vi "PH_Periodic_Sequencer.read DB.vi"(0 "i ref in":refnum<vi>, 5 "error in (no error)":errorcluster) -> (14 "i ref out":refnum<vi>, 19 "error out":errorcluster)   [LabVIEW 2009]
doc: "This VI reads out information from the database and stores it to own attributes."
uses:
  PH_Periodic_Sequencer.lvlib
  CSCore/BaseProcess/BaseProcess.lvlib
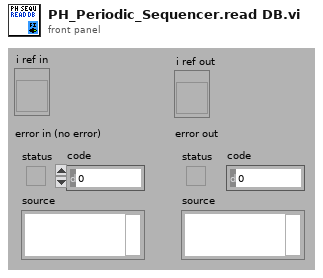
[diagram p1: front panel]
types:
  T1 = typedef "BaseProcess.lvlib/BaseProcess.i attribute.ctl" = cluster{"EventStatus":string, "EventError":i32, "PresetEvtWatchD":i32, "PresetPdcWatchD":i32, "EventTimeout":i32, "PeriodicInterval":i32, "Interface":string[], "Address":string[], "Special":string[], "PeriodicError":i32, "PeriodicStatus":string, "SuperProc":string, "Descriptors":T2[], "CaseRef":refnum<vi>, "PdcRef":refnum<vi>, "Thread Ref":refnum<vi>, "eventErrorID":i32, "eventStatusID":i32, "periodicErrorID":i32, "periodicStatusID":i32, "pdcCtrID":i32}
  T2 = typedef "BaseProcess.lvlib/BaseProcess.descriptor definition.ctl" = cluster{"selector":string, "descriptor":T3}
  T3 = typedef "BaseProcess.lvlib/BaseProcess.descriptor string definition.ctl" = string
  T4 = typedef "PH_Periodic_Sequencer.lvlib/PH_Periodic_Sequencer.i attribute.ctl" = cluster{"GUI Refs":cluster{"Main Off":refnum<vi>, "Start":refnum<vi>, "Ready":refnum<vi>, "Sequencer SM State":refnum<vi>, "Interval [sec]":refnum<vi>, "Wanted Shots":refnum<vi>, "Delivered Shots":refnum<vi>}, "PU Info":cluster{"Instancename":string, "State":T5, "linked":bool}[], "GUI Manager Path":string, "Sequencer":cluster{"Instancename":string, "linked?":bool, "R2S?":bool, "SM State":string}, "Run?":bool, "Interval [sec]":dbl, "PU State Refs":refnum<vi>[], "Wanted Shots":i32, "Delivered Shots":i32}
  T5 = typedef "Status.ctl" = i16
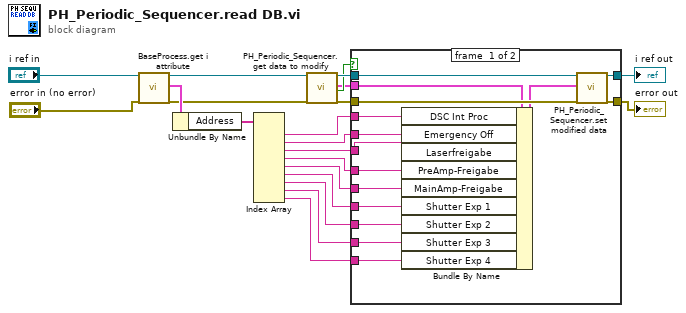
[diagram p0: block diagram]
diagram:
  n1 = call "BaseProcess.get i attribute.vi"("i ref in"="i ref in", "error in (no error)"="error in (no error)") -> ("i ref out"=w10:refnum<vi>, "i attribute"=w13:T1, "error out"=w11:errorcluster)  [unwired: 15 in]
  n2 = Unbundle By Name(w13) -> ("Address"=w12:string[])
  n3 = Index Array(array=w12) -> (element #1=w9:string, element #2=w8:string, element #3=w7:string, element #4=w6:string, element #5=w5:string, element #6=w4:string, element #7=w3:string, element #8=w2:string, element #9=w1:string)  [unwired: 9 in]
  n4 = call "PH_Periodic_Sequencer.get data to modify.vi"("i ref in"=w10, "error in (no error)"=w11) -> ("i ref out"=w21:refnum<vi>, "i attribute"=w16:T4, "timed out"=w17:bool, "error out"=w19:errorcluster)  [unwired: 14 in]
  n5 = case shown="False" w17 {
    tunnel: w21 -> [w36 w38]
    tunnel: [w35 w38] -> w20
    tunnel: w19 -> [w34 w37]
    tunnel: [w33 w37] -> w18
    tunnel: w16 -> [w32 _]
    tunnel: w9 -> [w30 _]
    tunnel: w8 -> [w29 _]
    tunnel: w7 -> [w28 _]
    tunnel: w6 -> [w27 _]
    tunnel: w5 -> [w26 _]
    tunnel: w4 -> [w25 _]
    tunnel: w3 -> [w24 _]
    tunnel: w2 -> [w23 _]
    tunnel: w1 -> [w22 _]
    frame #0 {
      n6 = Bundle By Name(cluster=w32, "DSC Int Proc"=w30, "Emergency Off"=w29, "Laserfreigabe"=w28, "PreAmp-Freigabe"=w27, "MainAmp-Freigabe"=w26, "Shutter Exp 1"=w25, "Shutter Exp 2"=w24, "Shutter Exp 3"=w23, "Shutter Exp 4"=w22) -> (w31:T4)
      n7 = call "PH_Periodic_Sequencer.set modified data.vi"("i ref in"=w36, "i attribute"=w31, "error in (no error)"=w34) -> ("i ref out"=w35:refnum<vi>, "error out"=w33:errorcluster)  [unwired: 15 in]
    }
    frame #1 {
    }
  }
  "i ref out" <- w20
  "error out" <- w18
